vi "Individual Sector ROIs.vi"(9 "right annulus":T2={"Center X"=929, "Center Y"=663, "Inner Radius"=200, "Outer Radius"=405, "Start Angle"=90.0, "End Angle"=180.0} {"End Angle" format="%.2f"; "Start Angle" format="%.2f"; "Center X" scale=0.0..1024.0}, 10 "left annulus":T2={"Center X"=929, "Center Y"=663, "Inner Radius"=200, "Outer Radius"=405, "Start Angle"=90.0, "End Angle"=180.0} {"End Angle" format="%.2f"; "Start Angle" format="%.2f"; "Center X" scale=0.0..1024.0}, 11 "Number of Sectors":u8=16) -> (3 "Sector ROIs":T1[](array[typedef]) {"Contours"."Type" items=["No Selection", "Point", "Line", "Rectangle", "Oval", "Polygon", "Freehand Region", "Annulus", "Unused2", "Unused3", "Broken Line", "Freehand Line", "Rotated Rectangle"]})   [LabVIEW 2013]
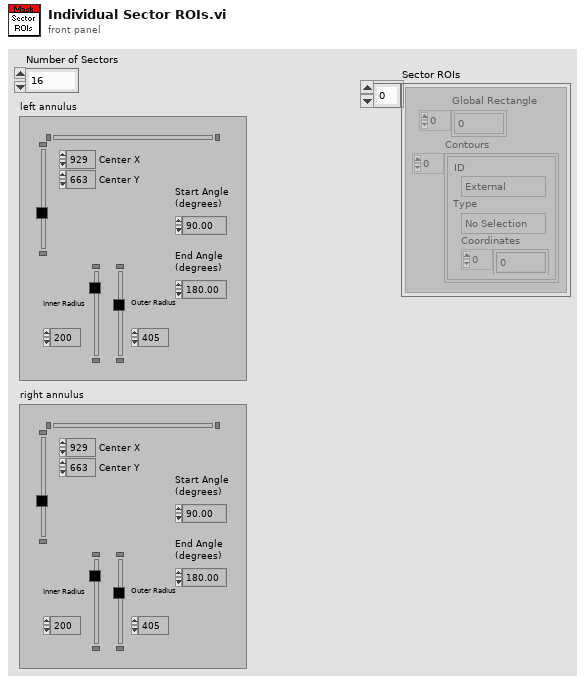
[diagram p1: front panel]
types:
  T1 = typedef "ROI Descriptor" = cluster{"Global Rectangle":i32[], "Contours":cluster{"ID":enum32{"External", "Internal"}, "Type":u32, "Coordinates":i32[]}[]}
  T2 = typedef "IMAQ Circle" = cluster{"Center X":i32, "Center Y":i32, "Inner Radius":i32, "Outer Radius":i32, "Start Angle":dbl, "End Angle":dbl}
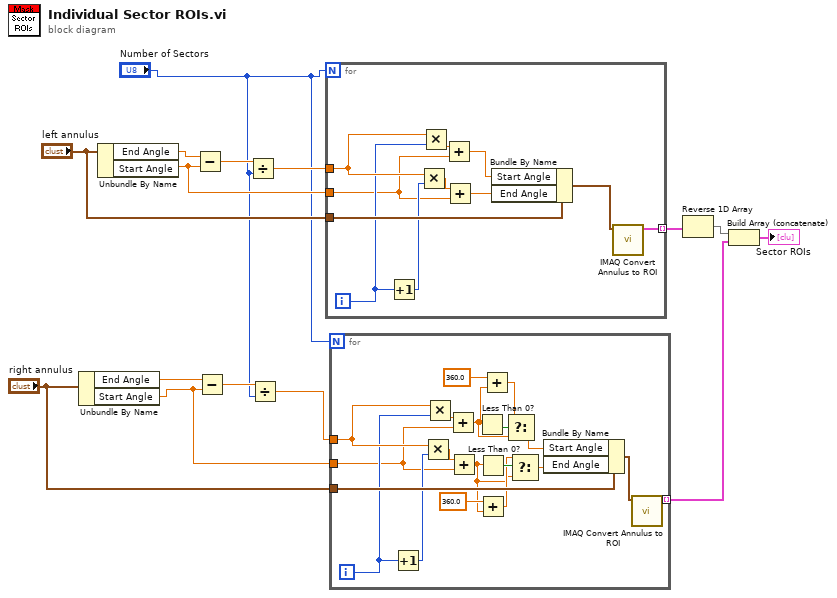
[diagram p0: block diagram]
diagram:
  n1 = Unbundle By Name("right annulus") -> ("End Angle"=w8:dbl, "Start Angle"=w5:dbl)
  n2 = Unbundle By Name("left annulus") -> ("End Angle"=w15:dbl, "Start Angle"=w12:dbl)
  n3 = Subtract(x=w15, y=w12) -> (x-y=w14:dbl)
  n4 = Subtract(x=w8, y=w5) -> (x-y=w9:dbl)
  n5 = Divide(x=w14, y="Number of Sectors") -> (x/y=w11:dbl)
  n6 = Divide(x=w9, y="Number of Sectors") -> (x/y=w7:dbl)
  n7 = for {
    N: "Number of Sectors" -> [_]
    tunnel: "left annulus" -> [w26]
    tunnel: w12 -> [w17]
    tunnel: w11 -> [w20]
    tunnel: [w21] -> w10 mode=indexing
    i -> [w19]
    n8 = Increment(x=w19) -> (x+1=w25:i32)
    n9 = Multiply(x=w20, y=w25) -> (x*y=w24:dbl)
    n10 = Multiply(x=w20, y=w19) -> (x*y=w18:dbl)
    n11 = Add(x=w18, y=w17) -> (x+y=w16:dbl)
    n12 = Add(x=w24, y=w17) -> (x+y=w23:dbl)
    n13 = Bundle By Name(cluster=w26, "Start Angle"=w16, "End Angle"=w23) -> (w22:T2)
    n14 = call "IMAQ Convert Annulus to ROI"("Annulus"=w22) -> ("ROI Descriptor"=w21:T1)  [unwired: 8 in, 1 out]
  }
  n15 = for {
    N: "Number of Sectors" -> [_]
    tunnel: "right annulus" -> [w45]
    tunnel: w5 -> [w38]
    tunnel: w7 -> [w41]
    tunnel: [w42] -> w3 mode=indexing
    i -> [w40]
    n16 = Increment(x=w40) -> (x+1=w44:i32)
    n17 = Multiply(x=w41, y=w44) -> (x*y=w43:dbl)
    n18 = Multiply(x=w41, y=w40) -> (x*y=w39:dbl)
    n19 = Add(x=w39, y=w38) -> (x+y=w32:dbl)
    n20 = Add(x=w43, y=w38) -> (x+y=w27:dbl)
    n21 = Less Than 0?(x=w32) -> (x < 0?=w35:bool)
    n22 = Less Than 0?(x=w27) -> (x < 0?=w31:bool)
    n23 = Add(x=360.0, y=w27) -> (x+y=w28:dbl)
    n24 = Add(x=360.0, y=w32) -> (x+y=w33:dbl)
    n25 = Select(t=w33, s=w35, f=w32) -> (s? t:f=w36:dbl)
    n26 = Select(t=w28, s=w31, f=w27) -> (s? t:f=w30:dbl)
    n27 = Bundle By Name(cluster=w45, "Start Angle"=w36, "End Angle"=w30) -> (w37:T2)
    n28 = call "IMAQ Convert Annulus to ROI"("Annulus"=w37) -> ("ROI Descriptor"=w42:T1)  [unwired: 8 in, 1 out]
  }
  n29 = Reverse 1D Array(array=w10) -> (reversed array=w4:T1[])
  n30 = Build Array (concatenate)(w4, w3) -> (→"Sector ROIs":T1[])
